vi "Set filter.vi"(8 "error in (no error)":errorcluster, 10 "Filter Num":i32, 11 "VISA resource name":refnum<visa-resource-name>) -> (0 "error out":errorcluster, 3 "VISA resource name out":refnum<visa-resource-name>)   [LabVIEW 2018]
uses:
  Controls/ACK Comm.ctl
  cfcce4bb-a8ba-49ac-9cc4-3623a9850227.vi
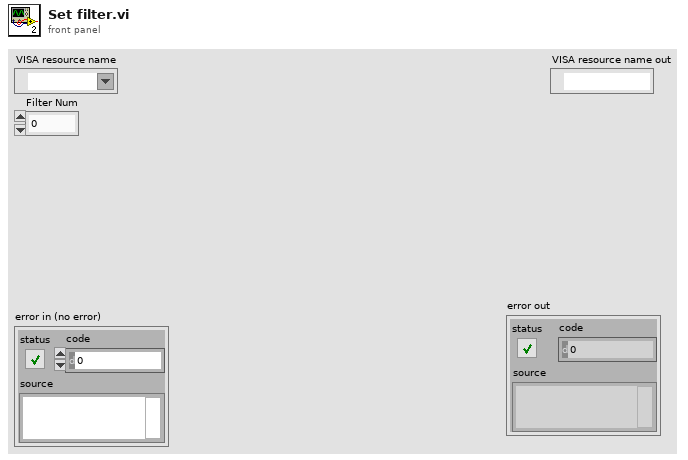
[diagram p1: front panel]
types:
  T1 = typedef "ACK Comm.ctl" = enum16{"Normal", "Filter Selection", "Shuuter Open", "Shutter Close"}
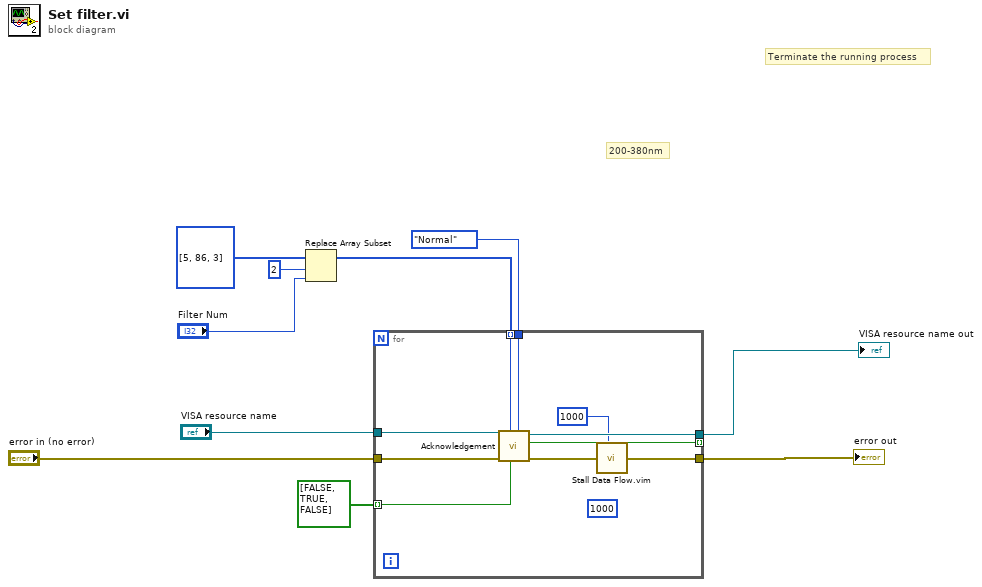
[diagram p0: block diagram]
diagram:
  # "200-380nm"
  # "Terminate the running process"
  n1 = Replace Array Subset(array=i32[] [5, 86, 3] ("Numeric"), new element="Filter Num", index=2) -> (w8:i32[])
  n2 = for {
    tunnel: w8 -> [w20] mode=indexing
    tunnel: ACK_Comm."Normal" ("Ack Comm") -> [w17]
    tunnel: [w16] -> _ mode=indexing
    tunnel: [w18] -> w1
    tunnel: [w14] -> w4
    tunnel: bool[] [FALSE, TRUE, FALSE] ("Inc") -> [w15] mode=indexing
    tunnel: "error in (no error)" -> [w12]
    tunnel: "VISA resource name" -> [w11]
    (unwired) u32 1000 ("milliseconds to wait")
    n3 = call "Acknowledgement.vi"(5:w17, "Inc"=w15, "Numeric"=w20, "error in (no error)"=w12, "VISA resource name"=w11) -> ("error out"=w19:errorcluster, "Connected?"=w16:bool, "VISA resource name out"=w18:refnum<visa-resource-name>)  [unwired: 4 in]
    n4 = call "Stall Data Flow.vim"("value in"=w19, "milliseconds to wait"=u32 1000) -> ("value out"=w14:errorcluster)  [unwired: 1 out]
  }
  "error out" <- w4
  "VISA resource name out" <- w1
